vi "Tutorial 01.vi"() -> ()   [LabVIEW 2014]
panel:
  in  "b":dbl
  out "c":dbl
  in  "a":dbl
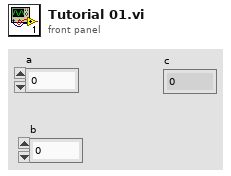
[diagram p1: front panel]
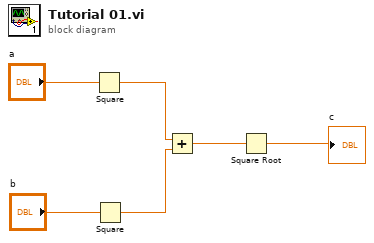
[diagram p0: block diagram]
diagram:
  n1 = Square(x="a") -> (x^2=w4:dbl)
  n2 = Square(x="b") -> (x^2=w3:dbl)
  n3 = Add(x=w4, y=w3) -> (x+y=w2:dbl)
  n4 = Square Root(x=w2) -> (sqrt(x)=→"c":dbl)
